vi "update.vi"(8 "error in (no error)":errorcluster, 10 "Model in":refnum<class "Model.lvclass">, 11 "EnabledState in":refnum<class "EnabledState.lvclass">) -> (0 "error out":errorcluster, 2 "Model out":refnum<class "Model.lvclass">, 3 "EnabledState out":refnum<class "EnabledState.lvclass">)   [LabVIEW 2016, in "EnabledState.lvclass"]
uses:
  EnabledState.lvclass
  Model/Model.lvclass
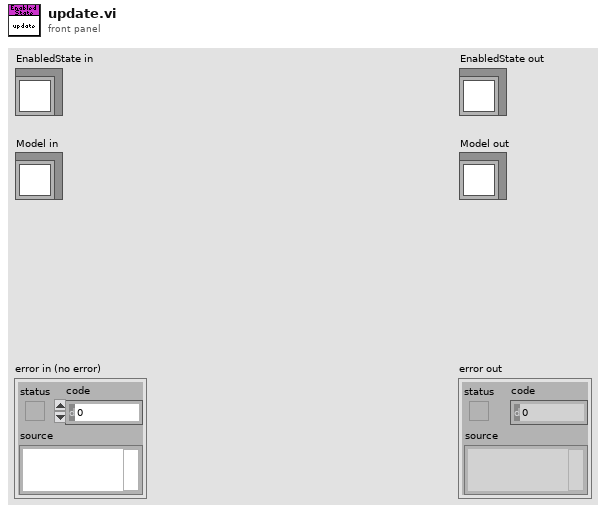
[diagram p1: front panel]
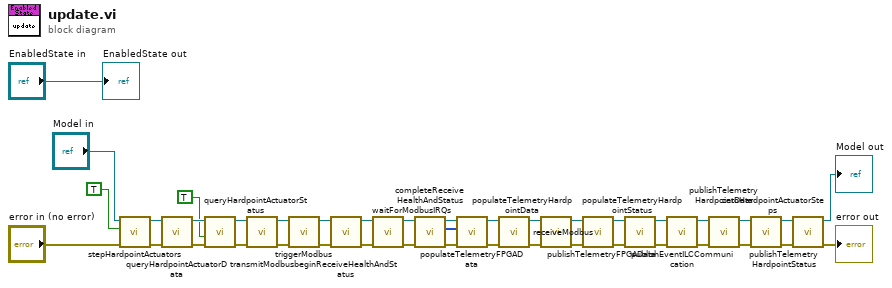
[diagram p0: block diagram]
diagram:
  n1 = call "stepHardpointActuators.vi"("error in (no error)"="error in (no error)", "WaitForTrigger"=TRUE, "Model in"="Model in") -> ("error out"=w6:errorcluster, "Model out"=w7:refnum<class "Model.lvclass">)  [unwired: 7 in]
  n2 = call "queryHardpointActuatorData.vi"("error in (no error)"=w6, "Model in"=w7) -> ("error out"=w22:errorcluster, "Model out"=w25:refnum<class "Model.lvclass">)  [unwired: 8 in]
  n3 = call "queryHardpointActuatorStatus.vi"("error in (no error)"=w22, "TriggerIRQ"=TRUE, "Model in"=w25) -> ("error out"=w23:errorcluster, "Model out"=w24:refnum<class "Model.lvclass">)  [unwired: 7 in]
  n4 = call "transmitModbus.vi"("error in (no error)"=w23, "Model in"=w24) -> ("error out"=w39:errorcluster, "Model out"=w40:refnum<class "Model.lvclass">)  [unwired: 8 in]
  n5 = call "triggerModbus.vi"("error in (no error)"=w39, "Model in"=w40) -> ("error out"=w37:errorcluster, "Model out"=w38:refnum<class "Model.lvclass">)  [unwired: 8 in]
  n6 = call "beginReceiveHealthAndStatus.vi"("error in (no error)"=w37, "Model in"=w38) -> ("error out"=w35:errorcluster, "Model out"=w36:refnum<class "Model.lvclass">)  [unwired: 8 in]
  n7 = call "waitForModbusIRQs.vi"("error in (no error)"=w35, "Model in"=w36) -> ("error out"=w34:errorcluster, "Model out"=w33:refnum<class "Model.lvclass">)  [unwired: 8 in]
  n8 = call "completeReceiveHealthAndStatus.vi"("error in (no error)"=w34, "Model in"=w33) -> ("error out"=w29:errorcluster, "Data"=w31:u32[], "Model out"=w28:refnum<class "Model.lvclass">)  [unwired: 7 in]
  n9 = call "populateTelemetryFPGAData.vi"("error in (no error)"=w29, "Data"=w31, "Model in"=w28) -> ("error out"=w26:errorcluster, "Model out"=w27:refnum<class "Model.lvclass">)  [unwired: 7 in]
  n10 = call "receiveModbus.vi"("error in (no error)"=w26, "Model in"=w27) -> ("error out"=w30:errorcluster, "Model out"=w32:refnum<class "Model.lvclass">)  [unwired: 8 in]
  n11 = call "populateTelemetryHardpointData.vi"("error in (no error)"=w30, "Model in"=w32) -> ("error out"=w19:errorcluster, "Model out"=w20:refnum<class "Model.lvclass">)  [unwired: 8 in]
  n12 = call "populateTelemetryHardpointStatus.vi"("error in (no error)"=w19, "Model in"=w20) -> ("error out"=w15:errorcluster, "Model out"=w16:refnum<class "Model.lvclass">)  [unwired: 8 in]
  n13 = call "publishTelemetryFPGAData.vi"("error in (no error)"=w15, "Model in"=w16) -> ("error out"=w12:errorcluster, "Model out"=w14:refnum<class "Model.lvclass">)  [unwired: 8 in]
  n14 = call "publishEventILCCommunication.vi"("error in (no error)"=w12, "Model in"=w14) -> ("error out"=w11:errorcluster, "Model out"=w13:refnum<class "Model.lvclass">)  [unwired: 8 in]
  n15 = call "publishTelemetryHardpointData.vi"("error in (no error)"=w11, "Model in"=w13) -> ("error out"=w17:errorcluster, "Model out"=w18:refnum<class "Model.lvclass">)  [unwired: 8 in]
  n16 = call "publishTelemetryHardpointStatus.vi"("error in (no error)"=w17, "Model in"=w18) -> ("error out"=w2:errorcluster, "Model out"=w4:refnum<class "Model.lvclass">)  [unwired: 8 in]
  n17 = call "zeroHardpointActuatorSteps.vi"("error in (no error)"=w2, "Model in"=w4) -> ("error out"=→"error out":errorcluster, "Model out"=→"Model out":refnum<class "Model.lvclass">)  [unwired: 8 in]
  "EnabledState out" <- "EnabledState in"
